vi "merFISH_main.vi"(0 "queue DAQ":refnum<queue>, 1 "queue ASI stage":refnum<queue>, 2 "queue ANDOR":refnum<queue>, 3 "queue piezo":refnum<queue>, 4 "merFISH path":path, 5 "error in":errorcluster, 6 "Laser list Refnum":refnum<vi>, 7 "Contrast":cluster{i32, i32}(slide)={16000, 0} scale=0.0..16000.0, 8 "Item Names":string[](array[string]), 9 "merFISH parameters":T2, 10 "Global parameters":T5={"405"=0.0, "488"=0.0, "561"=0.0, "641"=0.0, "BF"=0.0, "X"=0.0, "Y"=0.0, "Filter list"=1, "Exp time"=0.0, "Kinetic time"=0.0, "Gain"=0, "Step length (nm)"=0, "Total range (nm)"=0, "Scan illumination\n mode"=FALSE, "Dt (s)"=0, "# repetitions"=0} {"# repetitions" min=0; "Dt (s)" min=0 step=1; "Filter list" items=["ET665lp", "zet405/488/561/640m", "None", "None", "None", "None"]}, 11 "PID gains":T3={"proportional gain (Kc)"=2.0, "integral time (Ti, min)"=0.4, "derivative time (Td, min)"=0.0} {"derivative time (Td, min)" format="%.3f"; "integral time (Ti, min)" format="%.3f"; "proportional gain (Kc)" format="%.3f"}, 12 "RT image":T4, 13 "Treated image":T4, 14 "initialization cluster":cluster{"Ramp":dbl[], "Total # z steps":i32}) -> (19 "error merFISH":errorcluster)   [LabVIEW 2015]
uses:
  GLOBAL/Global_ABORT.vi
  CONTROLS/Q_MCL_piezo_element.ctl
  CONTROLS/Q_DAQ_element.ctl
  CONTROLS/Q_camera_element.ctl
  CONTROLS/Q_ASI_stage_element.ctl
  CONTROLS/Global parameters.ctl
  <vilib>/vision/Image Controls.llb/IMAQ Image.ctl
  CONTROLS/Q_main_element.ctl
panel:
  out "Numeric":i32
  out "error out":errorcluster
  in  "Illumination source":bool
  in  "Exp time (s)":sgl=0.05 format="%#_3g"
  out "Autofocus":bool
  in  "Abort merFISH":bool
  out "Number steps":i32
  out "Scan slider":u8(slide) scale=0.0..100.0
  out "XY positions":cluster{dbl[], dbl[]}[](graph)
  out "ROI manager":i32(listbox)
  out "Intensity":cluster{sgl, sgl}(slide) scale=0.0..16000.0
  out "Image":T4(plugin-control)
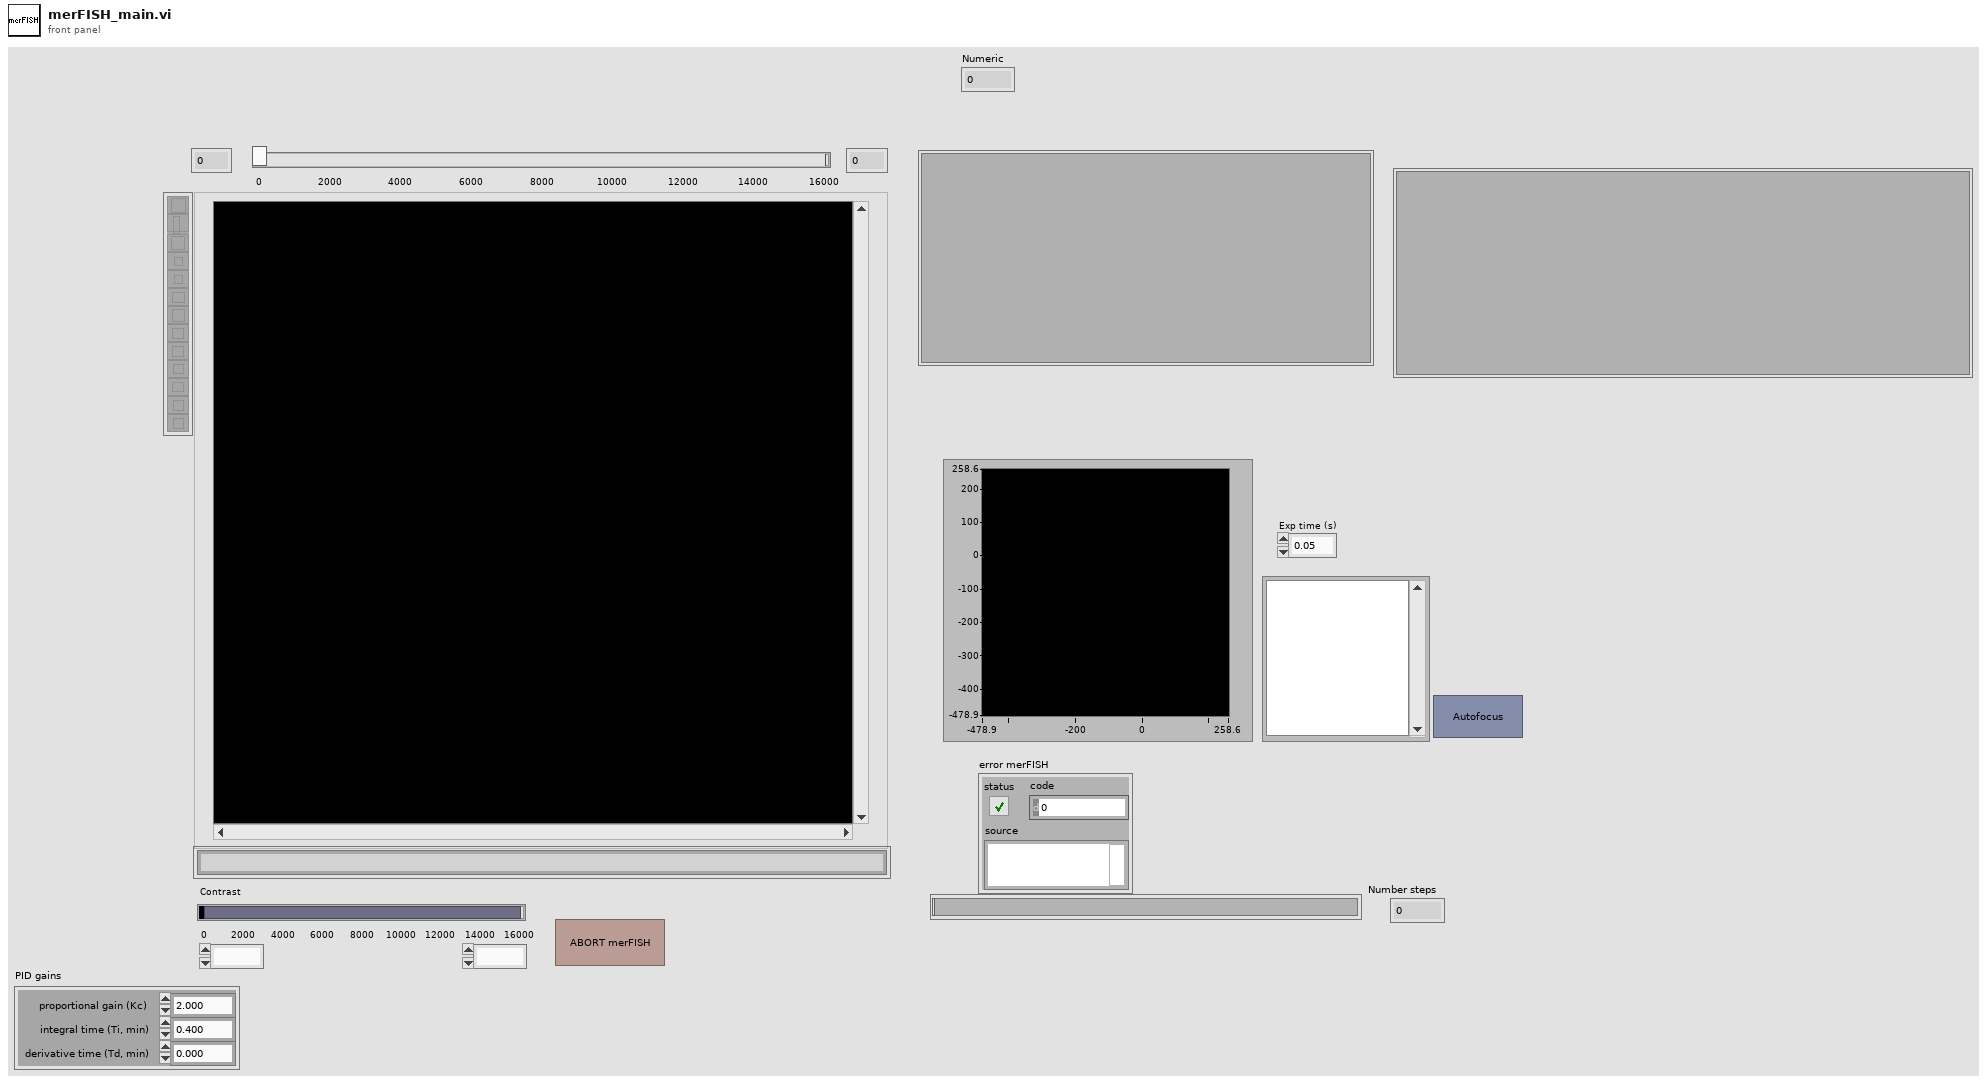
[diagram p1: front panel]
types:
  T1 = typedef "Q_main_element.ctl" = cluster{"variant":variant, "Instruction":enum16{"Main_idle", "Main_initialize", "Main_initialize_TDMS", "Main_initialize_Queue", "Main_error", "Main_DAQ_initialization_results", "Main_ASI_initialization_results", "Main_Piezo_initialization_results", "Main_Valve_initialization_results", "Main_Pump_initialization_results", "Main_CAMERA_initialization_results", "Main_DAQ_error", "Main_ASI_error", "Main_Piezo_error", "Main_CAMERA_error", "Main_Valve_error", "Main_Pump_error", "Main_start_acquiring", "Main_not_acquiring", "Main_acquiring", "Main_stop_acquiring", "Main_change_exposure", "Main_change_z_scan_parameters", "Main_define_ROI", "Main_read_kinetic_time", "Main_cooler", "Main_read_temperature", "Main_save_XY", "Main_load_XY", "Main_discard_XY", "Main_move_to_XY", "Main_measure_QPD", "Main_autofocus_calibration", "Main_save_PID", "Main_change_H_valve_position", "Main_two_way_valve", "Main_save_movie", "Main_init_single_scan", "Main_single_scan", "Main_stop_single_scan", "Main_merFISH_illumination_parameters", "Main_merFISH_buffer_probe_list", "Main_merFISH_injections_procedure", "Main_merFISH_save_setpoint", "Main_merFISH_DAPI_parameters", "Main_merFISH_Brightfield_parameters", "Main_merFISH_init", "Main_merFISH_resume", "Main_merFISH_start_autofocus", "Main_merFISH_open_close_valve_merFISH", "Main_merFISH_open_close_valve_photobleaching", "Main_merFISH_hybridization", "Main_merFISH_move_to_ROI", "Main_merFISH_wait_stabilization", "Main_merFISH_scan_laser", "Main_merFISH_scan_brightfield", "Main_merFISH_photobleaching_injection", "Main_merFISH_photobleaching", "Main_merFISH_save", "Main_merFISH_send_email", "Main_merFISH_close", "Main_TL_define_parameters", "Main_TL_reset_parameters", "Main_TL_init", "Main_TL_start_autofocus", "Main_TL_move_to_ROI", "Main_TL_wait_for_stabilization", "Main_TL_scan", "Main_TL_wait_cycle_end", "Main_TL_close", "Main_STOP"}}
  T2 = cluster{"XY positions":dbl[][], "Laser lines array":dbl[][], "merFISH init":cluster{"Autofocus calibrated":bool, "Autofocus setpoint defined":bool, "Laser defined":bool, "ROI defined":bool}, "QPD":cluster{"X":dbl, "Y":dbl, "intensity":dbl}, "Ramp":dbl[], "Task list":T1[], "Total # z steps":i32}
  T3 = cluster{"proportional gain (Kc)":dbl, "integral time (Ti, min)":dbl, "derivative time (Td, min)":dbl}
  T4 = typedef "IMAQ Image.ctl" = refnum<image>
  T5 = typedef "Global parameters.ctl" = cluster{"405":dbl, "488":dbl, "561":dbl, "641":dbl, "BF":dbl, "X":dbl, "Y":dbl, "Filter list":u16, "Exp time":sgl, "Kinetic time":sgl, "Gain":i32, "Step length (nm)":u32, "Total range (nm)":u32, "Scan illumination\n mode":bool, "Dt (s)":i32, "# repetitions":i32}
  T6 = typedef "Q_MCL_piezo_element.ctl" = cluster{"variant":variant, "Instruction":enum16{"Piezo_idle", "Piezo_initialize", "Piezo_error", "Piezo_security_stop", "Piezo_read_z", "Piezo_move_z", "Piezo_keyboard_move", "Piezo_close_autofocus_calibration_ramp", "Piezo_change_init_state", "Piezo_init_autofocus", "Piezo_init_autofocus_merFISH_TL", "Piezo_autofocus", "Piezo_autofocus_merFISH_TL", "Piezo_stop_autofocus", "Piezo_stop_autofocus_merFISH_TL", "Piezo_autofocus_lost", "Piezo_resume_autofocus_merFISH_TL", "Piezo_check_z_position_merFISH_TL", "Piezo_init_ramp", "Piezo_move_z_ramp", "Piezo_close_ramp", "Piezo_close_merFISH", "Piezo_init_TL", "Piezo_close_ramp_TL", "Piezo_close_TL", "Piezo_stop"}}
  T7 = cluster{"Maximal Value":sgl, "Minimal Value":sgl}
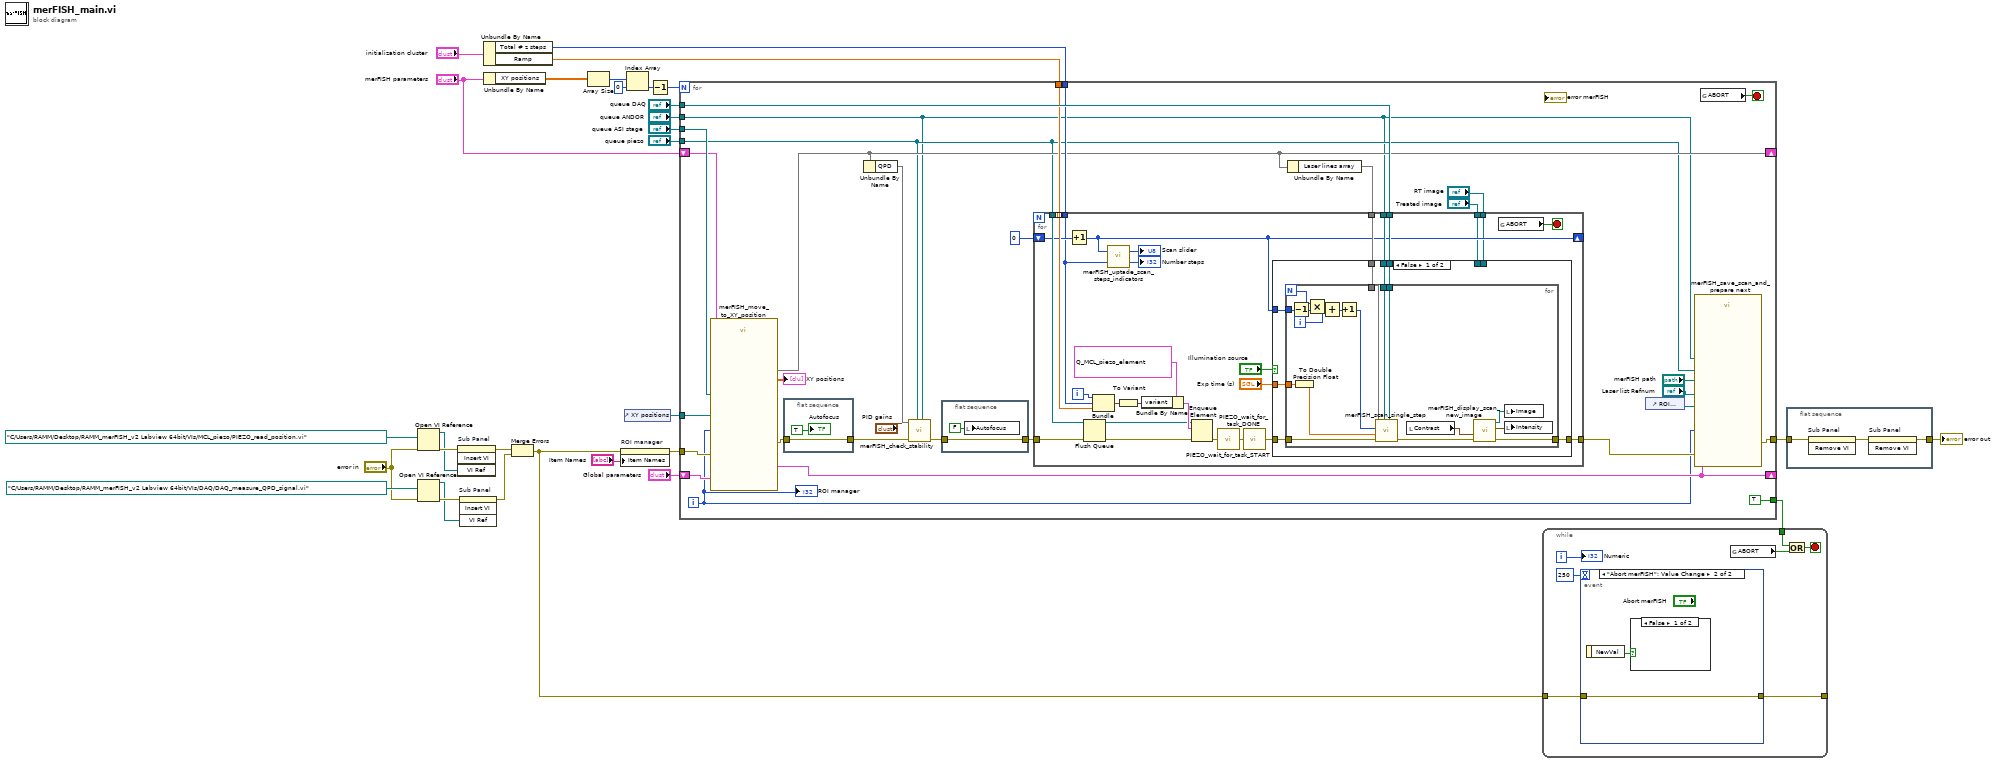
[diagram p0: block diagram]
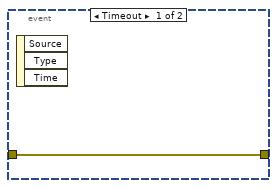
[diagram p2: hidden frame]
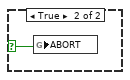
[diagram p3: hidden frame]
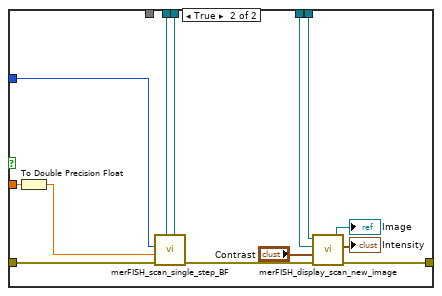
[diagram p4: hidden frame]
diagram:
  n1 = Open VI Reference(vi path=path "C:/Users/RAMM/Desktop/RAMM_merFISH_v2 Labview 64bit/VIs/MCL_piezo/PIEZO_read_position.vi", error in (no error)="error in") -> (vi reference=w23:refnum<vi>, error out=w27:errorcluster)  [unwired: 4 in]
  n2 = Open VI Reference(vi path=path "C:/Users/RAMM/Desktop/RAMM_merFISH_v2 Labview 64bit/VIs/DAQ/DAQ_measure_QPD_signal.vi", error in (no error)="error in") -> (vi reference=w8:refnum<vi>, error out=w25:errorcluster)  [unwired: 4 in]
  n3 = invoke on="Sub Panel" class="SubPnl" method="Insert VI"(error in=w27, "VI Ref"=w23) -> (error out=w26:errorcluster)  [unwired: 2 in, 3 out]
  n4 = invoke on="Sub Panel" class="SubPnl" method="Insert VI"(error in=w25, "VI Ref"=w8) -> (error out=w24:errorcluster)  [unwired: 2 in, 3 out]
  n5 = Unbundle By Name("initialization cluster") -> ("Total # z steps"=w6:i32, "Ramp"=w10:dbl[])
  n6 = Unbundle By Name("merFISH parameters") -> ("XY positions"=w19:dbl[][])
  n7 = Merge Errors(w26, w24) -> (w5:errorcluster)
  n8 = Array Size(array=w19) -> (size(s)=w20:i32[])
  n9 = property on="ROI manager" class="LstBox (strict)"(error in=w5, "Item Names"="Item Names") -> (error out=w4:errorcluster)  [unwired: 1 in, 1 out]
  n10 = control-ref of="XY positions"() -> (w16:refnum<vi>)
  n11 = Index Array(array=w20, index=0) -> (element=w22:i32)
  n12 = Decrement(x=w22) -> (x-1=w18:i32)
  n13 = for {
    N: w18 -> [_]
    tunnel: w4 -> [w60]
    tunnel: [w50] -> w9
    shift-right: [w54] -> _
    shift-left: "Global parameters" -> [w61]
    shift-right: [w40] -> _
    shift-left: "merFISH parameters" -> [w45]
    tunnel: w16 -> [w59]
    tunnel: "queue DAQ" -> [w56]
    tunnel: "queue ANDOR" -> [w38]
    tunnel: "queue ASI stage" -> [w57]
    tunnel: "queue piezo" -> [w39]
    tunnel: w10 -> [w55]
    tunnel: w6 -> [w49]
    tunnel: [TRUE] -> w2
    i -> [w41]
    stop <- w42 stop-if-true
    n14 = call "merFISH_move_to_XY_position.vi"("ROI #"=w41, "Global parameters"=w61, "queue ASI stage"=w57, 9:w59, "error in"=w60, "XY positions"=w45) -> ("Global parameters out"=w54:T5, "error out"=w34:errorcluster, 2:w40, "XY positions"=→"XY positions":dbl[][])  [unwired: 2 in]
    n15 = flat-sequence {
      tunnel: w34 -> [w64]
      tunnel: [w64] -> w33
      frame #0 {
        "Autofocus" <- TRUE ("Autofocus")
      }
    }
    n16 = Unbundle By Name(w40) -> ("QPD"=w37)
    n17 = call "merFISH_check_stability.vi"("queue ANDOR"=w38, "queue piezo"=w39, "error in"=w33, 10:"PID gains", 11:w37) -> ("error out"=w32:errorcluster)  [unwired: 6 in]
    n18 = flat-sequence {
      tunnel: w32 -> [w63]
      tunnel: [w63] -> w31
      frame #0 {
        n19 = local write "Autofocus"(FALSE ("Autofocus")) -> ()
      }
    }
    n20 = Unbundle By Name(w40) -> ("Laser lines array"=w47)
    n21 = for {
      tunnel: w56 -> [w74]
      tunnel: w55 -> [w82] mode=indexing
      tunnel: w39 -> [w83]
      tunnel: w38 -> [w75]
      tunnel: w31 -> [w84]
      tunnel: w49 -> [w73]
      shift-right: [w70] -> _
      shift-left: 0 -> [w80]
      tunnel: w47 -> [w77]
      tunnel: "Treated image" -> [w69]
      tunnel: "RT image" -> [w68]
      tunnel: [w67] -> w46
      i -> [w81]
      stop <- w66 stop-if-true
      n22 = Increment(x=w80) -> (x+1=w70:i32)
      n23 = Flush Queue(queue=w83, error in (no error)=w84) -> (queue out=w87:refnum<queue>, error out=w88:errorcluster)  [unwired: 1 out]
      n24 = Bundle(w81, "Total # z steps"=w73, w82) -> (w92:cluster{i32, "Total # z steps":i32, dbl})  [unwired: 1 in]
      n25 = call "merFISH_uptade_scan_steps_indicators.vi"("Total # steps"=w73, "scan step"=w70) -> ("scan step"=→"Number steps":i32, "slider"=→"Scan slider":u8)
      n26 = To Variant(anything=w92) -> (Variant=w86:variant)
      n27 = Bundle By Name(cluster=T6 {"variant"=variant, "Instruction"=enum."Piezo_move_z_ramp"} ("Q_MCL_Piezo"), "variant"=w86) -> (w89:T6)
      n28 = Enqueue Element(queue=w87, element=w89, error in (no error)=w88) -> (error out=w90:errorcluster)  [unwired: 1 in, 2 out]
      n29 = call "PIEZO_wait_for_task_START.vi"("error in"=w90) -> ("error out"=w91:errorcluster)
      n30 = call "PIEZO_wait_for_task_DONE.vi"("error in"=w91) -> ("error out"=w79:errorcluster)
      n31 = case shown="False" "Illumination source" {
        tunnel: w79 -> [w98 w124]
        tunnel: w77 -> [w99 _]
        tunnel: w70 -> [w97 w120]
        tunnel: "Exp time (s)" -> [w96 w122]
        tunnel: w75 -> [w95 w119]
        tunnel: w74 -> [w94 w118]
        tunnel: w69 -> [_ w130]
        tunnel: w68 -> [_ w129]
        tunnel: [w93 w128] -> w67
        frame False {
          n32 = for {
            N -> [w112]
            tunnel: w99 -> [w109]
            tunnel: w98 -> [w117]
            tunnel: w97 -> [w113]
            tunnel: w96 -> [w108]
            tunnel: w95 -> [w106]
            tunnel: w94 -> [w105]
            tunnel: [w100] -> w93
            i -> [w111]
            n33 = Decrement(x=w113) -> (x-1=w116:i32)
            n34 = To Double Precision Float(number=w108) -> (double precision float=w107:dbl)
            n35 = Multiply(x=w112, y=w116) -> (x*y=w114:i32)
            n36 = Add(x=w114, y=w111) -> (x+y=w115:i32)
            n37 = Increment(x=w115) -> (x+1=w110:i32)
            n38 = call "merFISH_scan_single_step.vi"("queue DAQ"=w105, "queue sCMOS"=w106, "error in"=w117, "Pulse length Ton (s)"=w107, "image #"=w110, "Laser lines"=w109) -> ("error out"=w101:errorcluster)  [unwired: 5 in]
            n39 = local read "Contrast"() -> (w104:cluster{i32, i32})
            n40 = call "merFISH_display_scan_new_image.vi"("error in"=w101, "Image contrast"=w104) -> ("error out"=w100:errorcluster, "intensity range"=w103:T7, "Image Dst Out"=w102:T4)  [unwired: 3 in]
            n41 = local write "Image"(w102) -> ()
            n42 = local write "Intensity"(w103) -> ()
          }
        }
        frame True {
          n43 = To Double Precision Float(number=w122) -> (double precision float=w121:dbl)
          n44 = call "merFISH_scan_single_step_BF.vi"("queue DAQ"=w118, "queue sCMOS"=w119, "error in"=w124, "Pulse length Ton (s)"=w121, "image #"=w120) -> ("error out"=w123:errorcluster)  [unwired: 6 in]
          n45 = call "merFISH_display_scan_new_image.vi"("error in"=w123, "Image contrast"="Contrast", "Treated image"=w130, "Real time image"=w129) -> ("error out"=w128:errorcluster, "intensity range"=→"Intensity":T7, "Image Dst Out"=→"Image":T4)  [unwired: 1 in]
        }
      }
      n46 = global read "Global_ABORT.vi" "ABORT"() -> (w66:bool)
    }
    n47 = control-ref of="ROI manager"() -> (w53:refnum<vi>)
    n48 = call "merFISH_save_scan_and_prepare next.vi"("merFISH path cluster"="merFISH path", "queue CAMERA"=w38, "queue piezo"=w39, "error in"=w46, "Global parameters"=w54, "ROI list Refnum"=w53, "Laser list Refnum"="Laser list Refnum", "Data"=w41) -> ("error out"=w50:errorcluster)  [unwired: 3 in]
    n49 = global read "Global_ABORT.vi" "ABORT"() -> (w42:bool)
    "ROI manager" <- w41
  }
  n50 = while {
    tunnel: w5 -> [w136]
    tunnel: [w135] -> _
    tunnel: w2 -> [w133]
    i -> [w134]
    stop <- w131 stop-if-true
    n51 = event shown="[1] \"Abort merFISH\": Value Change" {
      selector: _ -> [_ _]
      dyn-events: _ -> [_ _]
      timeout: 250 -> [_ _]
      tunnel: w136 -> [w138 w140]
      tunnel: [w138 w140] -> w135
      event Timeout {
        n52 = event-data() -> ()  [unwired: 1 in, 3 out]
      }
      event "Abort merFISH": Value Change {
        n53 = event-data() -> ("NewVal"=w139:bool)  [unwired: 1 in]
        n54 = case shown="False" w139 {
          selector: w139 -> [_ w141]
          frame False {
          }
          frame True {
            n55 = global write "Global_ABORT.vi" "ABORT"(w141) -> ()
          }
        }
      }
    }
    n56 = global read "Global_ABORT.vi" "ABORT"() -> (w132:bool)
    n57 = Or(x=w133, y=w132) -> (x .or. y?=w131:bool)
    "Numeric" <- w134
  }
  n58 = flat-sequence {
    tunnel: w9 -> [w144]
    tunnel: [w142] -> w7
    frame #0 {
      n59 = invoke on="Sub Panel" class="SubPnl" method="Remove VI"(error in=w144) -> (error out=w143:errorcluster)  [unwired: 2 in, 2 out]
      n60 = invoke on="Sub Panel" class="SubPnl" method="Remove VI"(error in=w143) -> (error out=w142:errorcluster)  [unwired: 2 in, 2 out]
    }
  }
  "error out" <- w7
